vi "Init.vi"(8 "error in":errorcluster, 11 "Acquire Continuous Waveform Configuration in":refnum<class "DS1054 Base CFG.lvclass">) -> (0 "error out":errorcluster, 3 "Acquire Continuous Waveform Configuration out":refnum<class "DS1054 Base CFG.lvclass">)   [LabVIEW 2023, in "RIGOL DS1054Z.lvlib" / "DS1054 Base CFG.lvclass"]
uses:
  DS1054 Base CFG.lvclass
  Configuration Base/Configuration Base.lvclass/Configuration Base.ctl
  Scope/Scope VISA/Configuration/Scope VISA CFG.lvclass/Scope VISA CFG.ctl
  a845dea6-c2f2-4e03-ac8d-35208e94dd6c.vi
  <vilib>/JDP Science/JSONtext/Find Item.vi
  <vilib>/JDP Science/JSONtext/Next JSON Value.vi
  <vilib>/JDP Science/JSONtext/String Subset.vi
  <vilib>/JDP Science/JSONtext/Parsing/Advance past next JSON Value (inlined COPY).vi
  <vilib>/JDP Science/JSONtext/Parsing/Advance past whitespace.vi
  <vilib>/JDP Science/JSONtext/Parsing/Advance past String.vi
  <vilib>/JDP Science/JSONtext/Parsing/Advance past Number.vi
  <vilib>/JDP Science/JSONtext/Parsing/Advance past Line Ending.vi
  <vilib>/JDP Science/JSONtext/Parsing/Parse Full Path or Item Name.vi
  <vilib>/JDP Science/JSONtext/Parsing/Advance past Array.vi
  <vilib>/JDP Science/JSONtext/Parsing/Advance past Object.vi
  <vilib>/JDP Science/JSONtext/support/Error Cluster From Code.vi
  <vilib>/JDP Science/JSONtext/Offset/Find Item Locations by Path.vi
  <vilib>/JDP Science/JSONtext/JSON text to Variant.vi
  <vilib>/Utility/error.llb/Error Cluster From Error Code.vi
  <vilib>/JDP Science/JSONtext/LVClass Serializer/JSONtext LVClass Serializer.lvclass
  <vilib>/ErrorRing/Error Ring.xnode
  <instrlib>/RIGOL-DS1054Z-LabVIEW/RIGOL DS1054Z Driver.lvlib
  Configuration Base/Configuration Base.lvclass
  Scope/Scope VISA/Configuration/Scope VISA CFG.lvclass
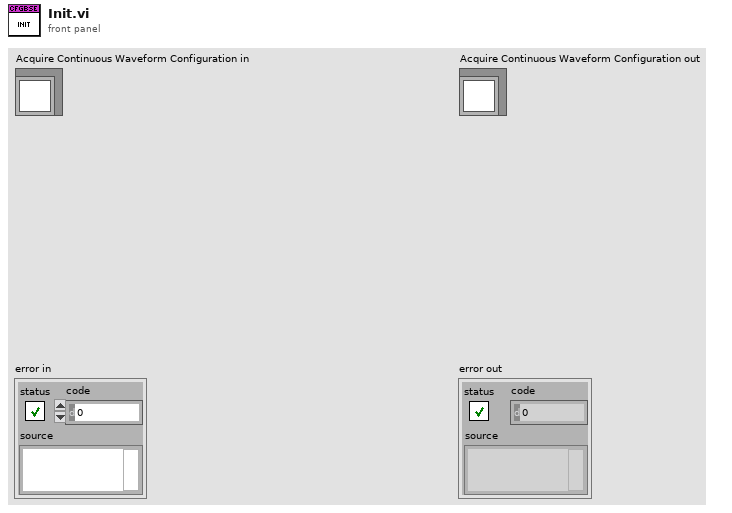
[diagram p1: front panel]
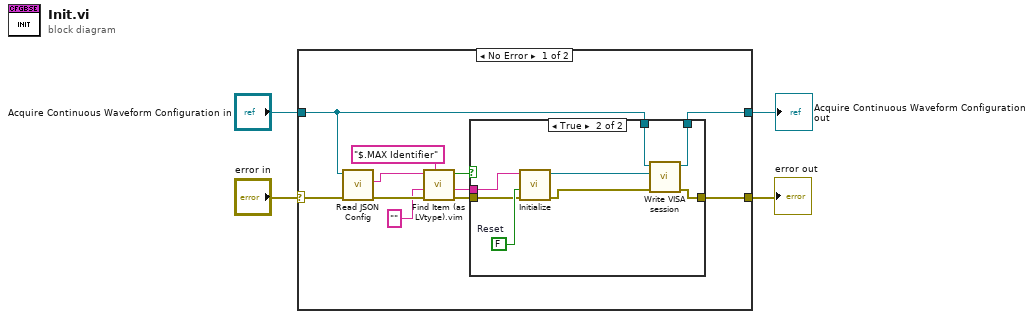
[diagram p0: block diagram]
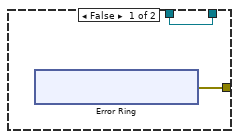
[diagram p2: hidden frame]
diagram:
  n1 = case shown="No Error" "error in" {
    selector: "error in" -> [w13 w32]
    tunnel: "Acquire Continuous Waveform Configuration in" -> [w5 w31]
    tunnel: [w15 w31] -> w3
    tunnel: [w14 w32] -> w1
    frame No Error {
      n2 = call "Read JSON Config.vi"("error in"=w13, "object in"=w5) -> ("error out"=w11:errorcluster, "<JSON>Config"=w12:string)  [unwired: 7 in, 1 out]
      n3 = call "Find Item (as LVtype).vim"("$Path or Item Name"="$.MAX Identifier", "error in (no error)"=w11, "Data Type and Default Value"="", "JSON"=w12) -> ("error out"=w6:errorcluster, "Data"=w8:string, "Found"=w7:bool)  [unwired: 4 in, 1 out]
      n4 = case shown="True" w7 {
        tunnel: [w16 w27] -> w15
        tunnel: [w17 w23] -> w14
        tunnel: w8 -> [_ w29]
        tunnel: w6 -> [_ w28]
        tunnel: w5 -> [w16 w26]
        frame False {
          n5 = xnode "Error Ring"() -> ("error out"=w17:errorcluster)
        }
        frame True {
          w30 = FALSE  # Reset
          n6 = call <instrlib>:"Initialize.vi"("error in (no error)"=w28, "Reset (True)"=w30, "VISA resource name"=w29) -> ("error out"=w24:errorcluster, "VISA resource name out"=w25:refnum<visa-resource-name>)  [unwired: 1 in, 6 out]
          n7 = call "Write VISA session.vi"("error in (no error)"=w24, "VISA session"=w25, "Scope VISA CFG in"=w26) -> ("error out"=w23:errorcluster, "Scope VISA CFG out"=w27:refnum<class "DS1054 Base CFG.lvclass">)  [unwired: 7 in]
        }
      }
    }
    frame Error {
    }
  }
  "error out" <- w1
  "Acquire Continuous Waveform Configuration out" <- w3
